vi "SplineHelp_GetCubicSpline_Calc2.vi"(8 "newWayPts":T1[](array[typedef]), 9 "dy-in":dbl[](array[numeric]), 11 "dx-in":dbl[](array[numeric])) -> (1 "dy-out":dbl[](array[numeric]), 3 "dx-out":dbl[](array[numeric]))   [LabVIEW 2019, in "Trajectory_Library.lvlib"]
doc: "Internal routine called by: SplineHelp_getCubicSplinesFromControlVectors.vi"
uses:
  Trajectory_Library.lvlib
  TRANSLATION2D.ctl
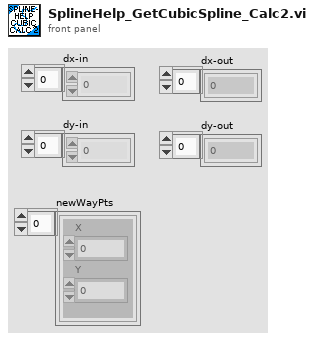
[diagram p1: front panel]
types:
  T1 = typedef "Trajectory_Library.lvlib/TRANSLATION2D.ctl" = cluster{"X":dbl, "Y":dbl}
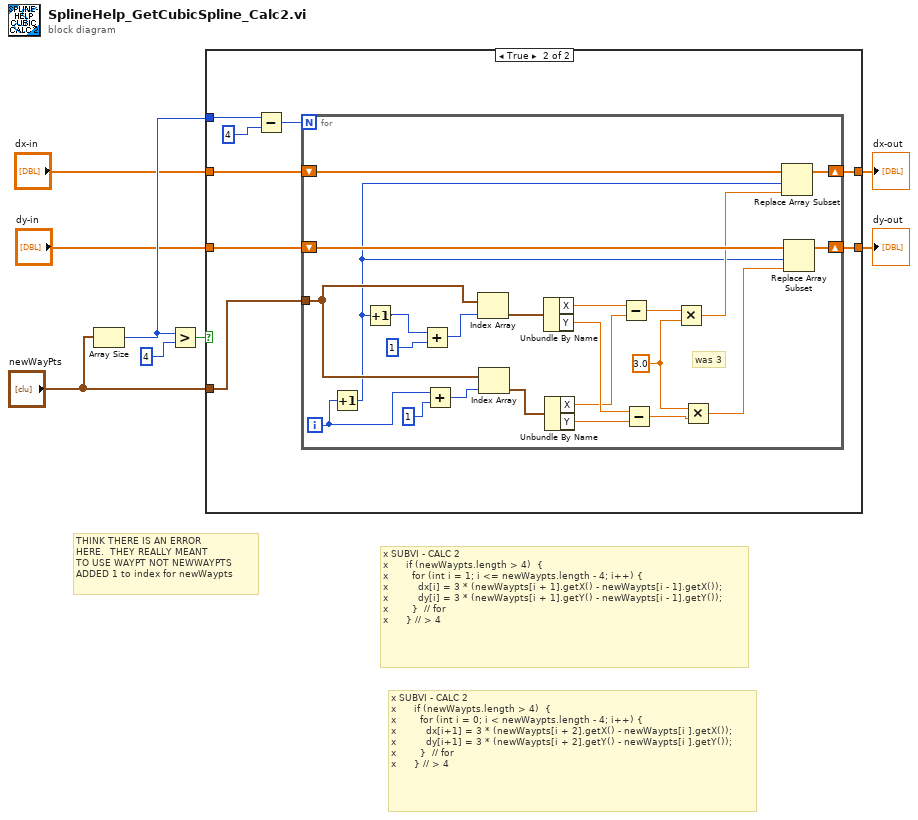
[diagram p0: block diagram]
diagram:
  # "THINK THERE IS AN ERROR\nHERE.  THEY REALLY MEANT\nTO USE WAYPT NOT NEWWAYPTS\nADDED 1 to index for newWaypts"
  # "x SUBVI - CALC 2\nx      if (newWaypts.length > 4)  { \nx        for (int i = 0; i < newWaypts.length - 4; i++) {\nx          dx[i+1] = 3 * (newWaypts[i + 2].getX() - newWaypts[i ].getX());\nx          dy[i+1] = 3 * (newWaypts[i + 2].getY() - newWaypts[i ].getY());\nx        }  // for\nx      } // > 4"
  # "x SUBVI - CALC 2\nx      if (newWaypts.length > 4)  { \nx        for (int i = 1; i <= newWaypts.length - 4; i++) {\nx          dx[i] = 3 * (newWaypts[i + 1].getX() - newWaypts[i - 1].getX());\nx          dy[i] = 3 * (newWaypts[i + 1].getY() - newWaypts[i - 1].getY());\nx        }  // for\nx      } // > 4"
  n1 = Array Size(array="newWayPts") -> (size(s)=w8:i32)
  n2 = Greater?(x=w8, y=4) -> (0:w1:bool)
  n3 = case shown="True" w1 {
    tunnel: w8 -> [_ w17]
    tunnel: "dy-in" -> [w9 w14]
    tunnel: "dx-in" -> [w10 w15]
    tunnel: "newWayPts" -> [_ w13]
    tunnel: [w9 w12] -> w5
    tunnel: [w10 w11] -> w4
    frame False {
    }
    frame True {
      n4 = Subtract(x=w17, y=4) -> (x-y=w16:i32)
      n5 = for {
        N: w16 -> [_]
        shift-right: [w38] -> w11
        shift-left: w15 -> [w41]
        shift-right: [w39] -> w12
        shift-left: w14 -> [w40]
        tunnel: w13 -> [w29]
        i -> [w23]
        w35 = 3.0
        # "was 3"
        n6 = Increment(x=w23) -> (x+1=w25:i32)
        n7 = Increment(x=w25) -> (x+1=w24:i32)
        n8 = Add(x=w24, y=1) -> (x+y=w20:i32)
        n9 = Add(x=w23, y=1) -> (x+y=w19:i32)
        n10 = Index Array(array=w29, index=w20) -> (element=w28:T1)
        n11 = Index Array(array=w29, index=w19) -> (element=w27:T1)
        n12 = Unbundle By Name(w28) -> ("X"=w34:dbl, "Y"=w33:dbl)
        n13 = Unbundle By Name(w27) -> ("X"=w26:dbl, "Y"=w32:dbl)
        n14 = Subtract(x=w34, y=w26) -> (x-y=w37:dbl)
        n15 = Subtract(x=w33, y=w32) -> (x-y=w36:dbl)
        n16 = Multiply(x=w37, y=w35) -> (x*y=w31:dbl)
        n17 = Multiply(x=w35, y=w36) -> (x*y=w30:dbl)
        n18 = Replace Array Subset(array=w41, new element=w31, index=w25) -> (w38:dbl[])
        n19 = Replace Array Subset(array=w40, new element=w30, index=w25) -> (w39:dbl[])
      }
    }
  }
  "dy-out" <- w5
  "dx-out" <- w4
